vi "Controls to Commands.vi"(11 "Robot Controls":T2) -> (3 "Robot Commands":T1)   [LabVIEW 2015]
uses:
  Robot Controls.ctl
  Robot Commands.ctl
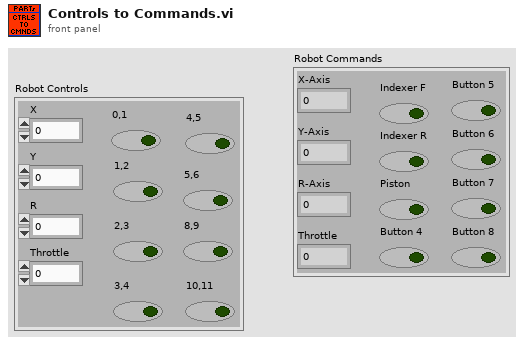
[diagram p1: front panel]
types:
  T1 = typedef "Robot Commands.ctl" = cluster{"X-Axis":dbl, "Y-Axis":dbl, "R-Axis":dbl, "Throttle":dbl, "Indexer F":bool, "Indexer R":bool, "Piston":bool, "Button 4":bool, "Button 5":bool, "Button 6":bool, "Button 7":bool, "Button 8":bool}
  T2 = typedef "Robot Controls.ctl" = cluster{"X":dbl, "Y":dbl, "R":dbl, "Throttle":dbl, "0,1":bool, "1,2":bool, "2,3":bool, "3,4":bool, "4,5":bool, "5,6":bool, "8,9":bool, "10,11":bool}
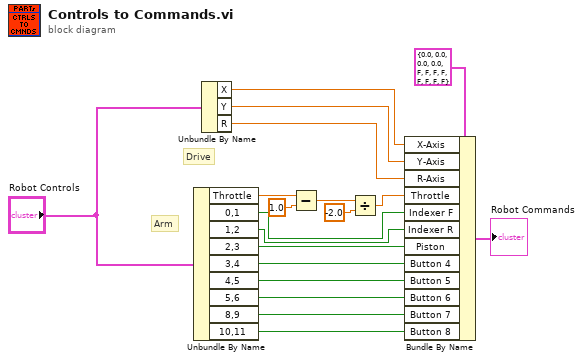
[diagram p0: block diagram]
diagram:
  # "Arm"
  # "Drive"
  n1 = Unbundle By Name("Robot Controls") -> ("Throttle"=w10:dbl, "0,1"=w12:bool, "1,2"=w13:bool, "2,3"=w14:bool, "3,4"=w15:bool, "4,5"=w16:bool, "5,6"=w17:bool, "8,9"=w18:bool, "10,11"=w19:bool)
  n2 = Unbundle By Name("Robot Controls") -> ("X"=w3:dbl, "Y"=w4:dbl, "R"=w5:dbl)
  n3 = Subtract(x=w10, y=1.0) -> (x-y=w9:dbl)
  n4 = Divide(x=w9, y=-2.0) -> (x/y=w11:dbl)
  n5 = Bundle By Name(cluster=T1 {"X-Axis"=0.0, "Y-Axis"=0.0, "R-Axis"=0.0, "Throttle"=0.0, "Indexer F"=FALSE, "Indexer R"=FALSE, "Piston"=FALSE, "Button 4"=FALSE, "Button 5"=FALSE, "Button 6"=FALSE, "Button 7"=FALSE, "Button 8"=FALSE} ("Robot Commands"), "X-Axis"=w3, "Y-Axis"=w4, "R-Axis"=w5, "Throttle"=w11, "Indexer F"=w12, "Indexer R"=w13, "Piston"=w14, "Button 4"=w15, "Button 5"=w16, "Button 6"=w17, "Button 7"=w18, "Button 8"=w19) -> (→"Robot Commands":T1)
